vi "Unregister Loggers.vi"(8 "error in (no error)":errorcluster) -> (0 "error out":errorcluster, 3 "failures info":T1[](array[typedef]) {"Log Record"."timestamp" format="%<%x %.3X>T"})   [LabVIEW 2018, in "GLog.lvlib"]
doc: "Unregister all currently registered loggers in the Registry."
uses:
  GLog.lvlib
  logger_class/Failure Information.ctl
  logger_class/Log Record.ctl
  logger_class/Internal Log Levels.ctl
  logger_class/Logger.lvclass
  registry/Registry.lvlib
panel:
  # "Connector Pane"
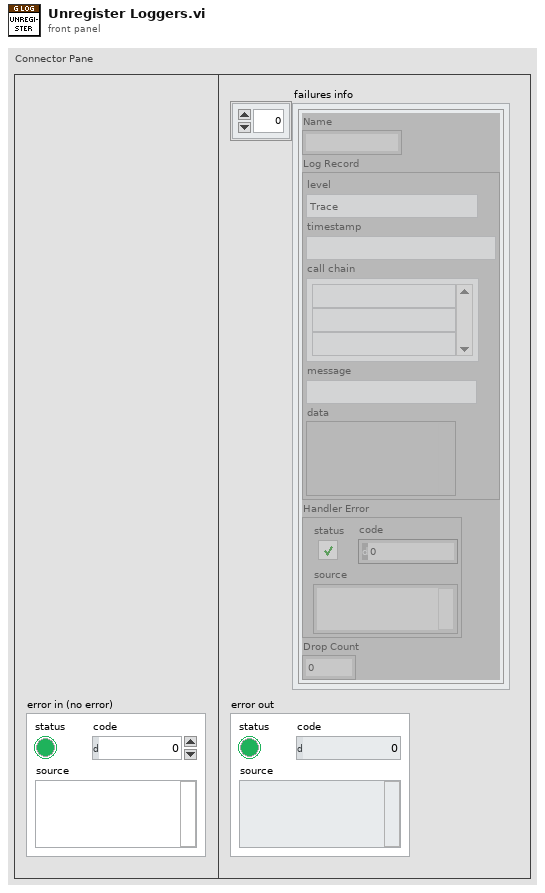
[diagram p1: front panel]
types:
  T1 = typedef "GLog.lvlib/Logger.lvclass/Failure Information.ctl" = cluster{"Name":string, "Log Record":T2, "Handler Error":errorcluster, "Drop Count":u32}
  T2 = typedef "GLog.lvlib/Logger.lvclass/Log Record.ctl" = cluster{"level":T3, "timestamp":timestamp, "call chain":string[], "message":string, "data":variant}
  T3 = typedef "GLog.lvlib/Logger.lvclass/Internal Log Levels.ctl" = enum16{"Trace", "Debug", "Info", "Warning", "Error", "Critical", "Internal"}
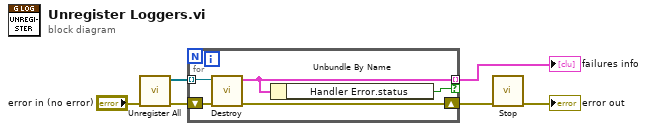
[diagram p0: block diagram]
diagram:
  n1 = call "Unregister All.vi"("error in (no error)"="error in (no error)") -> ("error out"=w3:errorcluster, "loggers"=w5:refnum<class "Logger.lvclass">[])  [unwired: 9 in]
  n2 = for {
    shift-right: [w10] -> w2
    shift-left: w3 -> [w11]
    tunnel: w5 -> [w9] mode=indexing
    tunnel: [w8] -> w6 mode=indexing if=w7
    n3 = call "Destroy.vi"("error in (no error)"=w11, "logger in"=w9) -> ("error out"=w10:errorcluster, "failure info"=w8:T1)  [unwired: 8 in]
    n4 = Unbundle By Name(w8) -> ("Handler Error.status"=w7:bool)
  }
  "failures info" <- w6
  n5 = call "Stop.vi"("error in (no error)"=w2) -> ("error out"=→"error out":errorcluster)  [unwired: 10 in]
